vi "Meta.vi"(10 "error in (no error)":errorcluster, 11 "Config Element in":refnum<class "Config Element.lvclass">) -> (2 "error out":errorcluster, 3 "Meta Data":T1[](array[typedef]))   [LabVIEW 2020, in "CDM-Config.lvlib" / "Config Element.lvclass"]
doc: "Returns all meta fields that are set on the element."
uses:
  Config Element.lvclass
  Meta Data.ctl
  CDM-Config.lvlib
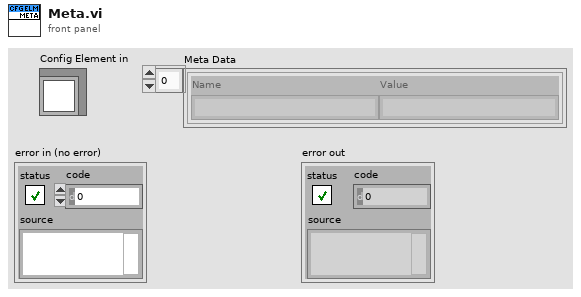
[diagram p1: front panel]
types:
  T1 = typedef "CDM-Config.lvlib/Meta Data.ctl" = cluster{"Name":string, "Value":string}
  T2 = typedef "CDM-Config.lvlib/Config Element.lvclass/Ref Data.ctl" = cluster{"Node Info":T3, "Owner":refnum<class>, "Changed":bool, "Name":string, "Value":string, "Meta Data":T1[]}
  T3 = typedef "CDM-Config.lvlib/Node Info.ctl" = cluster{"Index":i32, "Parent":i32, "Children":i32[]}
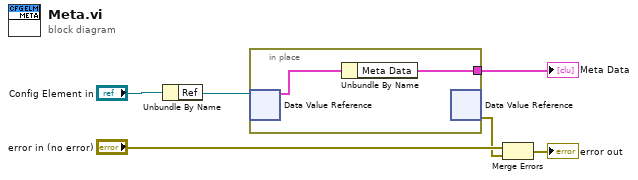
[diagram p0: block diagram]
diagram:
  n1 = Unbundle By Name("Config Element in") -> ("Ref"=w1:refnum<data-value>)
  n2 = in-place {
    in-place-border: [w7] -> w2
    n3 = in-place-dvr #1(w1) -> (w8:T2)  [unwired: 1 out]
    n4 = Unbundle By Name(w8) -> ("Meta Data"=w7:T1[])
    n5 = in-place-dvr #1() -> (w3:errorcluster)  [unwired: 1 in, 1 out]
  }
  "Meta Data" <- w2
  n6 = Merge Errors("error in (no error)", w3) -> (→"error out":errorcluster)
